vi "Swerve Drive.vi"(0 "X":dbl, 1 "Rot. Point X":dbl, 3 "Rot. Point Y":dbl, 5 "Y":dbl, 7 "Z":dbl, 11 "Error In":errorcluster, 12 "Robot Centric?":bool=TRUE, 13 "Autonomous?":bool, 14 "Yaw":dbl) -> (4 "Front Left Output":dbl, 6 "Front Right Output":dbl, 8 "Back Left Output":dbl, 10 "Back Right Output":dbl, 15 "Error Out":errorcluster)   [LabVIEW 2017]
uses:
  Public/Documents/Cross The Road Electronics/Phoenix-LabVIEW/Motor Controller/Controls/CTRE_Phoenix_MotorControl_ControlMode.ctl
  <vilib>/Rock Robotics/Network Tables/NT Read Number.vi
  <vilib>/Rock Robotics/Network Tables/NT Write Numeric Array.vi
panel:
  in  "Robot Length":dbl=33.5
  in  "Robot Width":dbl=28.5
  # "Swerve Drive Teleoperated Control\nFRC Team 34"
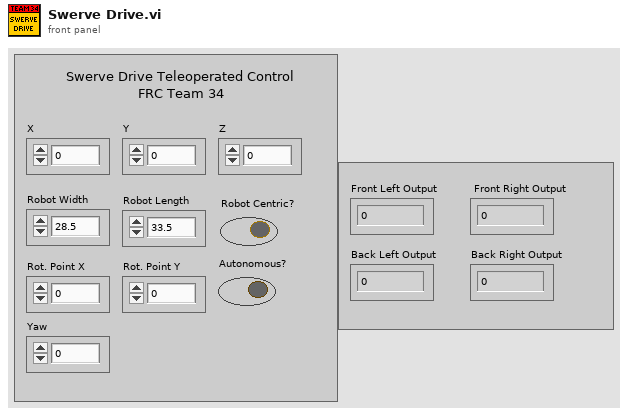
[diagram p1: front panel]
types:
  T1 = typedef "CTRE_Phoenix_MotorControl_ControlMode.ctl" = u16
  T2 = enum16{"Front Left", "Front Right", "Back Left", "Back Right"}
  T3 = typedef "WPI_MotorControlDeviceRef.ctl" = cluster{"DeviceStatus":errorcluster, "Type":T4, "PWM":cluster{"PWM Channel":T5, "DeadBand":T6}, "CAN":cluster{"Device Number":u8, "SetOutput VI Ref":variant, "GetOutput VI Ref":variant, "Enable VI Ref":variant, "Disable VI Ref":variant, "Data":variant}, "Invert":bool, "DIO PWM":cluster{"PWM \"Enable\" Channel":T5, "DIOChannel":T7, "PWM Rate":dbl}}
  T4 = typedef "WPI_MotorControlType.ctl" = enum16{"PWM", "CAN", "DIO PWM"}
  T5 = typedef "FPGA_DIOPWMChannel.ctl" = enum8{"PWM 0", "PWM 1", "PWM 2", "PWM 3", "PWM 4", "PWM 5", "PWM 6", "PWM 7", "PWM 8", "PWM 9", "PWM MXP 0", "PWM MXP 1", "PWM MXP 2", "PWM MXP 3", "PWM MXP 4", "PWM MXP 5", "PWM MXP 6", "PWM MXP 7", "PWM MXP 8", "PWM MXP 9", "Invalid"}
  T6 = typedef "WPI_PWMDeadband.ctl" = cluster{"Name":string, "maxPositivePwm":i32, "minPositivePwm":i32, "centerPwm":i32, "maxNegativePwm":i32, "minNegativePwm":i32, "angularRange":u16}
  T7 = typedef "FPGA_DIOChannel.ctl" = enum8{"DIO 0", "DIO 1", "DIO 2", "DIO 3", "DIO 4", "DIO 5", "DIO 6", "DIO 7", "DIO 8", "DIO 9", "DIO MXP 0", "DIO MXP 1", "DIO MXP 2", "DIO MXP 3", "DIO MXP 4", "DIO MXP 5", "DIO MXP 6", "DIO MXP 7", "DIO MXP 8", "DIO MXP 9", "DIO MXP 10", "DIO MXP 11", "DIO MXP 12", "DIO MXP 13", "DIO MXP 14", "DIO MXP 15", "SPI Port CS1", "SPI Port CS2", "SPI Port CS3", "SPI Port MISO", "SPI Port MOSI", "Invalid"}
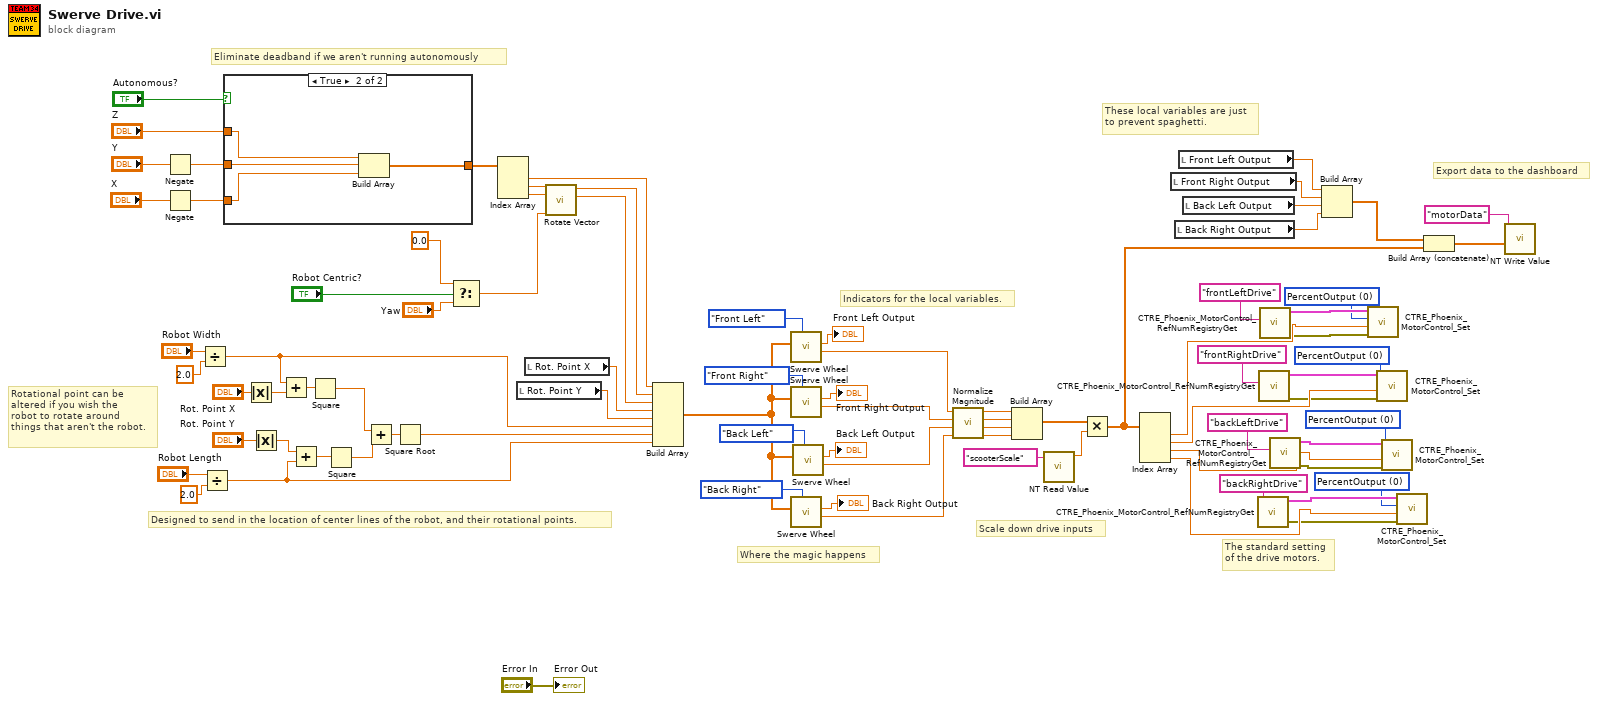
[diagram p0: block diagram]
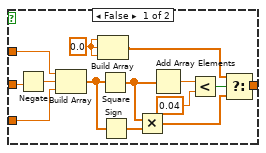
[diagram p2: hidden frame]
diagram:
  w9 = T1 0 items=["PercentOutput"=0, "Position"=1, "Velocity"=2, "Current"=3, "Follower"=5, "MotionProfile"=6, "MotionMagic"=7, "MotionMagicArc"=8, "MotionProfileArc"=10, "Disabled"=15] ("Control Mode")
  w10 = T1 0 items=["PercentOutput"=0, "Position"=1, "Velocity"=2, "Current"=3, "Follower"=5, "MotionProfile"=6, "MotionMagic"=7, "MotionMagicArc"=8, "MotionProfileArc"=10, "Disabled"=15] ("Control Mode")
  w11 = T1 0 items=["PercentOutput"=0, "Position"=1, "Velocity"=2, "Current"=3, "Follower"=5, "MotionProfile"=6, "MotionMagic"=7, "MotionMagicArc"=8, "MotionProfileArc"=10, "Disabled"=15] ("Control Mode")
  w12 = T1 0 items=["PercentOutput"=0, "Position"=1, "Velocity"=2, "Current"=3, "Follower"=5, "MotionProfile"=6, "MotionMagic"=7, "MotionMagicArc"=8, "MotionProfileArc"=10, "Disabled"=15] ("Control Mode")
  # "Export data to the dashboard"
  # "Indicators for the local variables."
  # "Rotational point can be \naltered if you wish the \nrobot to rotate around \nthings that aren't the robot."
  # "Scale down drive inputs"
  # "Eliminate deadband if we aren't running autonomously"
  # "These local variables are just \nto prevent spaghetti."
  # "Where the magic happens"
  # "The standard setting\nof the drive motors."
  # "Designed to send in the location of center lines of the robot, and their rotational points."
  n1 = Negate(x="Y") -> (-x=w30:dbl)
  n2 = Negate(x="X") -> (-x=w29:dbl)
  n3 = Divide(x="Robot Width", y=2.0) -> (x/y=w56:dbl)
  n4 = Divide(x="Robot Length", y=2.0) -> (x/y=w54:dbl)
  n5 = case shown="True" "Autonomous?" {
    tunnel: w30 -> [w87 w100]
    tunnel: [w86 w98] -> w82
    tunnel: "Z" -> [w85 w101]
    tunnel: w29 -> [w84 w99]
    frame False {
      w93 = 0.0 ("element")
      n6 = Negate(x=w87) -> (-x=w89:dbl)
      n7 = Build Array(w85, w89, w84) -> (w92:dbl[])
      n8 = Build Array(w93, w93, w93) -> (w94:dbl[])
      n9 = Square(x=w92) -> (x^2=w90:dbl[])
      n10 = Sign(1:w92) -> (0:w91:dbl[])
      n11 = Multiply(x=w90, y=w91) -> (x*y=w88:dbl[])
      n12 = Add Array Elements(numeric array=w90) -> (sum=w97:dbl)
      n13 = Less?(x=w97, y=0.04 ("x")) -> (x < y?=w95:bool)
      n14 = Select(t=w94, s=w95, f=w88) -> (s? t:f=w86:dbl[])
    }
    frame True {
      n15 = Build Array(w101, w100, w99) -> (w98:dbl[])
    }
  }
  n16 = Absolute Value(x="Rot. Point X") -> (abs(x)=w68:dbl)
  n17 = Absolute Value(x="Rot. Point Y") -> (abs(x)=w65:dbl)
  n18 = Add(x=w56, y=w68) -> (x+y=w67:dbl)
  n19 = Add(x=w65, y=w54) -> (x+y=w66:dbl)
  n20 = Square(x=w67) -> (x^2=w63:dbl)
  n21 = Square(x=w66) -> (x^2=w64:dbl)
  n22 = Add(x=w63, y=w64) -> (x+y=w62:dbl)
  n23 = Square Root(x=w62) -> (sqrt(x)=w55:dbl)
  n24 = Select(t=0.0, s="Robot Centric?", f="Yaw") -> (s? t:f=w75:dbl)
  n25 = Index Array(array=w82) -> (element #1=w61:dbl, element #2=w77:dbl, element #3=w76:dbl)  [unwired: 3 in]
  n26 = local read "Rot. Point Y"() -> (w57:dbl)
  n27 = local read "Rot. Point X"() -> (w58:dbl)
  n28 = call "Rotate Vector.vi"("Angle"=w75, "X"=w76, "Y"=w77) -> ("X'"=w59:dbl, "Y'"=w60:dbl)  [unwired: 7 in]
  n29 = Build Array(w61, w60, w59, w58, w57, w56, w55, w54) -> (w53:dbl[])
  n30 = call "Swerve Wheel.vi"("Wheel"=T2."Front Left", "Inputs"=w53) -> ("Speed"=w48:dbl, "Motor Output"=→"Front Left Output":dbl)  [unwired: 8 in]
  n31 = call "Swerve Wheel.vi"("Wheel"=T2."Front Right", "Inputs"=w53) -> ("Speed"=w47:dbl, "Motor Output"=→"Front Right Output":dbl)  [unwired: 8 in]
  n32 = call "Swerve Wheel.vi"("Wheel"=T2."Back Right", "Inputs"=w53) -> ("Speed"=w45:dbl, "Motor Output"=→"Back Right Output":dbl)  [unwired: 8 in]
  n33 = call "Swerve Wheel.vi"("Wheel"=T2."Back Left", "Inputs"=w53) -> ("Speed"=w46:dbl, "Motor Output"=→"Back Left Output":dbl)  [unwired: 8 in]
  n34 = call "Normalize Magnitude.vi"("D"=w45, "C"=w46, "B"=w47, "A"=w48) -> ("D'"=w41:dbl, "C'"=w42:dbl, "B'"=w43:dbl, "A'"=w44:dbl)  [unwired: 4 in]
  n35 = Build Array(w44, w43, w42, w41) -> (w40:dbl[])
  n36 = call-poly <vilib>:"NT Read Value.vi"("Name"="scooterScale") -> ("Numeric"=w38:dbl)  [unwired: 9 in, 1 out]
  n37 = Multiply(x=w40, y=w38) -> (x*y=w1:dbl[])
  n38 = Index Array(array=w1) -> (element #1=w23:dbl, element #2=w17:dbl, element #3=w14:dbl, element #4=w20:dbl)  [unwired: 4 in]
  n39 = local read "Front Right Output"() -> (w4:dbl)
  n40 = local read "Back Right Output"() -> (w2:dbl)
  n41 = local read "Front Left Output"() -> (w5:dbl)
  n42 = local read "Back Left Output"() -> (w3:dbl)
  n43 = call "CTRE_Phoenix_MotorControl_RefNumRegistryGet.vi"("refnum name"="backRightDrive") -> ("error out"=w19:errorcluster, "PhoenixMotorControlDevRef"=w21:T3)  [unwired: 9 in]
  n44 = call "CTRE_Phoenix_MotorControl_RefNumRegistryGet.vi"("refnum name"="frontRightDrive") -> ("error out"=w16:errorcluster, "PhoenixMotorControlDevRef"=w18:T3)  [unwired: 9 in]
  n45 = call "CTRE_Phoenix_MotorControl_RefNumRegistryGet.vi"("refnum name"="frontLeftDrive") -> ("error out"=w22:errorcluster, "PhoenixMotorControlDevRef"=w24:T3)  [unwired: 9 in]
  n46 = call "CTRE_Phoenix_MotorControl_RefNumRegistryGet.vi"("refnum name"="backLeftDrive") -> ("error out"=w13:errorcluster, "PhoenixMotorControlDevRef"=w15:T3)  [unwired: 9 in]
  n47 = Build Array(w5, w4, w3, w2) -> (w8:dbl[])
  n48 = call "CTRE_Phoenix_MotorControl_Set.vi"("error in (no error)"=w22, "Output"=w23, "Control Mode"=w12, "PhoenixMotorControlDevRef"=w24) -> ()  [unwired: 6 in, 2 out]
  n49 = call "CTRE_Phoenix_MotorControl_Set.vi"("error in (no error)"=w16, "Output"=w17, "Control Mode"=w11, "PhoenixMotorControlDevRef"=w18) -> ()  [unwired: 6 in, 2 out]
  n50 = call "CTRE_Phoenix_MotorControl_Set.vi"("error in (no error)"=w13, "Output"=w14, "Control Mode"=w10, "PhoenixMotorControlDevRef"=w15) -> ()  [unwired: 6 in, 2 out]
  n51 = call "CTRE_Phoenix_MotorControl_Set.vi"("error in (no error)"=w19, "Output"=w20, "Control Mode"=w9, "PhoenixMotorControlDevRef"=w21) -> ()  [unwired: 6 in, 2 out]
  n52 = Build Array (concatenate)(w8, w1) -> (w7:dbl[])
  n53 = call-poly <vilib>:"NT Write Value.vi"("Numeric Array"=w7, "Name"="motorData") -> ()  [unwired: 9 in, 1 out]
  "Error Out" <- "Error In"
